vi "Harry_kane_home_use.vi"() -> ()   [LabVIEW 2013]
uses:
  <vilib>/vision/NI_Vision_Development_Module.lvlib
panel:
  out "appended array":cluster{"X":sgl, "Y":sgl}[](array[cluster])
  out "Pitch Image":T1(plugin-control)
  out "Player Position Pixels":dbl[][](array[numeric])
  out "Puck position pixels":dbl[][](array[numeric])
  out "Player Array From Reference":dbl[][](array[numeric])
  out "Puck Array From Reference":dbl[][](array[numeric])
  in  "Calibrate":bool
  out "Binary":T1(plugin-control)
  out "Histogram":T2(graph)
  out "Image in":T1(plugin-control)
  in  "Stop":bool
  in  "Capture image":bool
  out "Calibrated":T1(plugin-control)
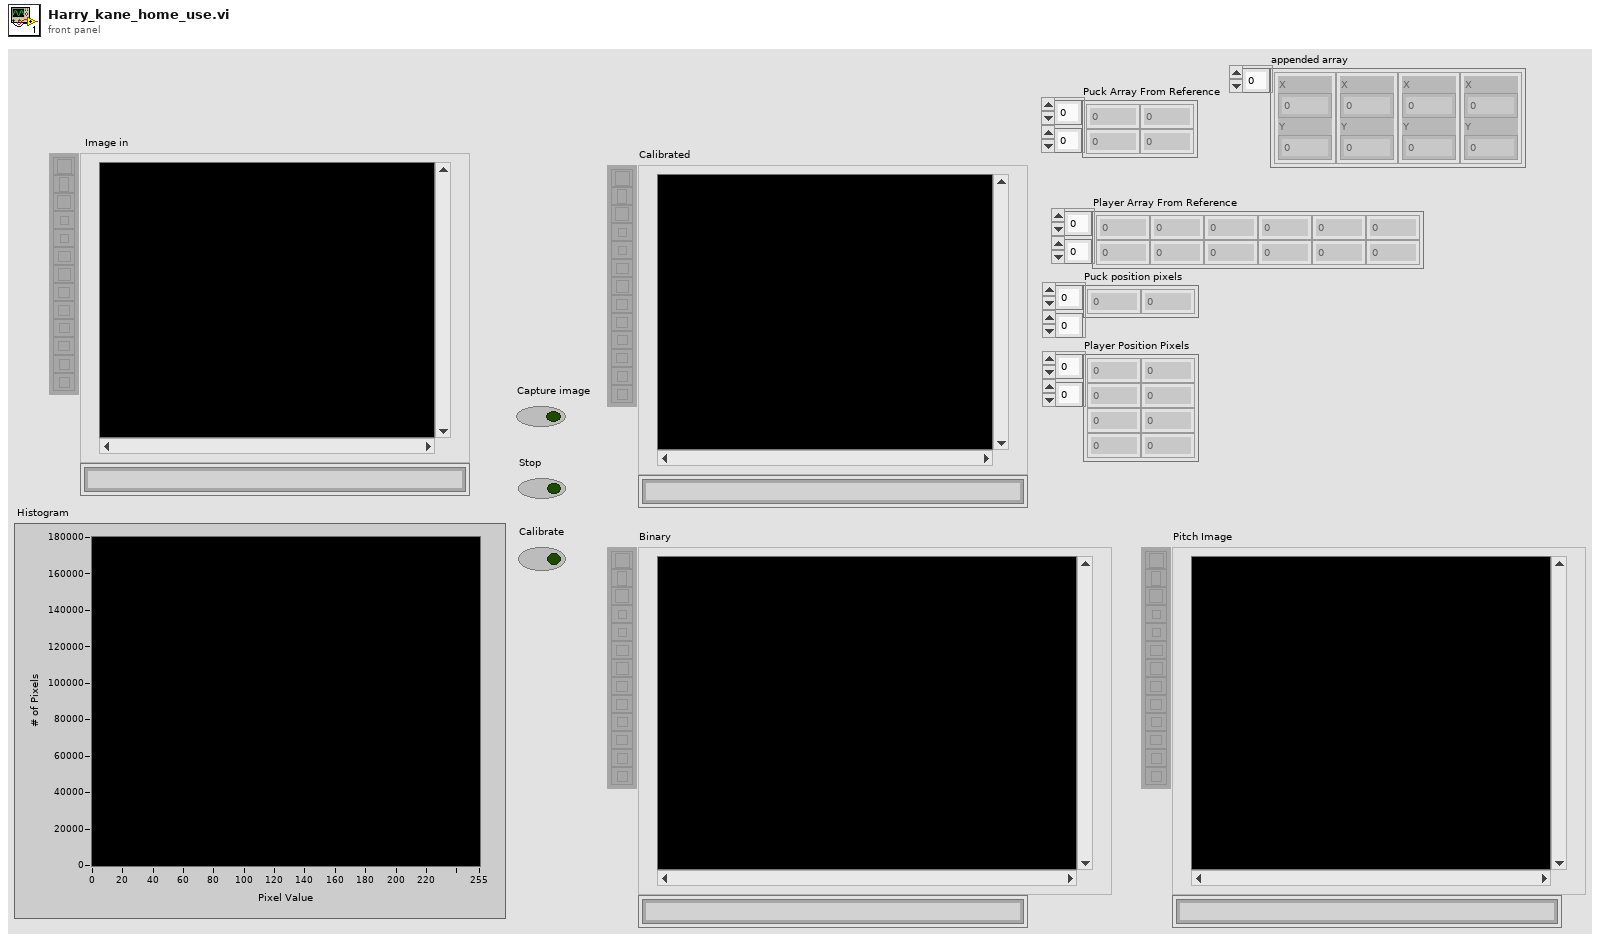
[diagram p1: front panel]
types:
  T1 = typedef "IMAQ Image.ctl" = refnum<image>
  T2 = cluster{"Starting Value":sgl, "Incremental Value":sgl, "Histogram":u32[]}
  T3 = typedef "Image Type" = u32
  T4 = cluster{"Point1 (Pixels)":cluster{"X":sgl, "Y":sgl}, "Point2 (Pixels)":cluster{"X":sgl, "Y":sgl}, "Point1 (Real-World)":cluster{"X":sgl, "Y":sgl}, "Point2 (Real-World)":cluster{"X":sgl, "Y":sgl}, "Angle (Pixel)":dbl, "Angle (Real-World)":dbl, "Score":dbl, "Straightness":dbl, "Average SNR (db)":dbl, "Calibration Valid":bool}
  T5 = cluster{"Start Point":cluster{"X":sgl, "Y":sgl}, "End Point":cluster{"X":sgl, "Y":sgl}, "Length":dbl, "Orientation":dbl, "Score":dbl}[]
  T6 = cluster{"Point1 (Pixels)":cluster{"X":sgl, "Y":sgl}, "Point2 (Pixels)":cluster{"X":sgl, "Y":sgl}}
  T7 = cluster{"Start Point":cluster{"X":sgl, "Y":sgl}, "End Point":cluster{"X":sgl, "Y":sgl}, "Length":dbl, "Orientation":dbl, "Score":dbl}
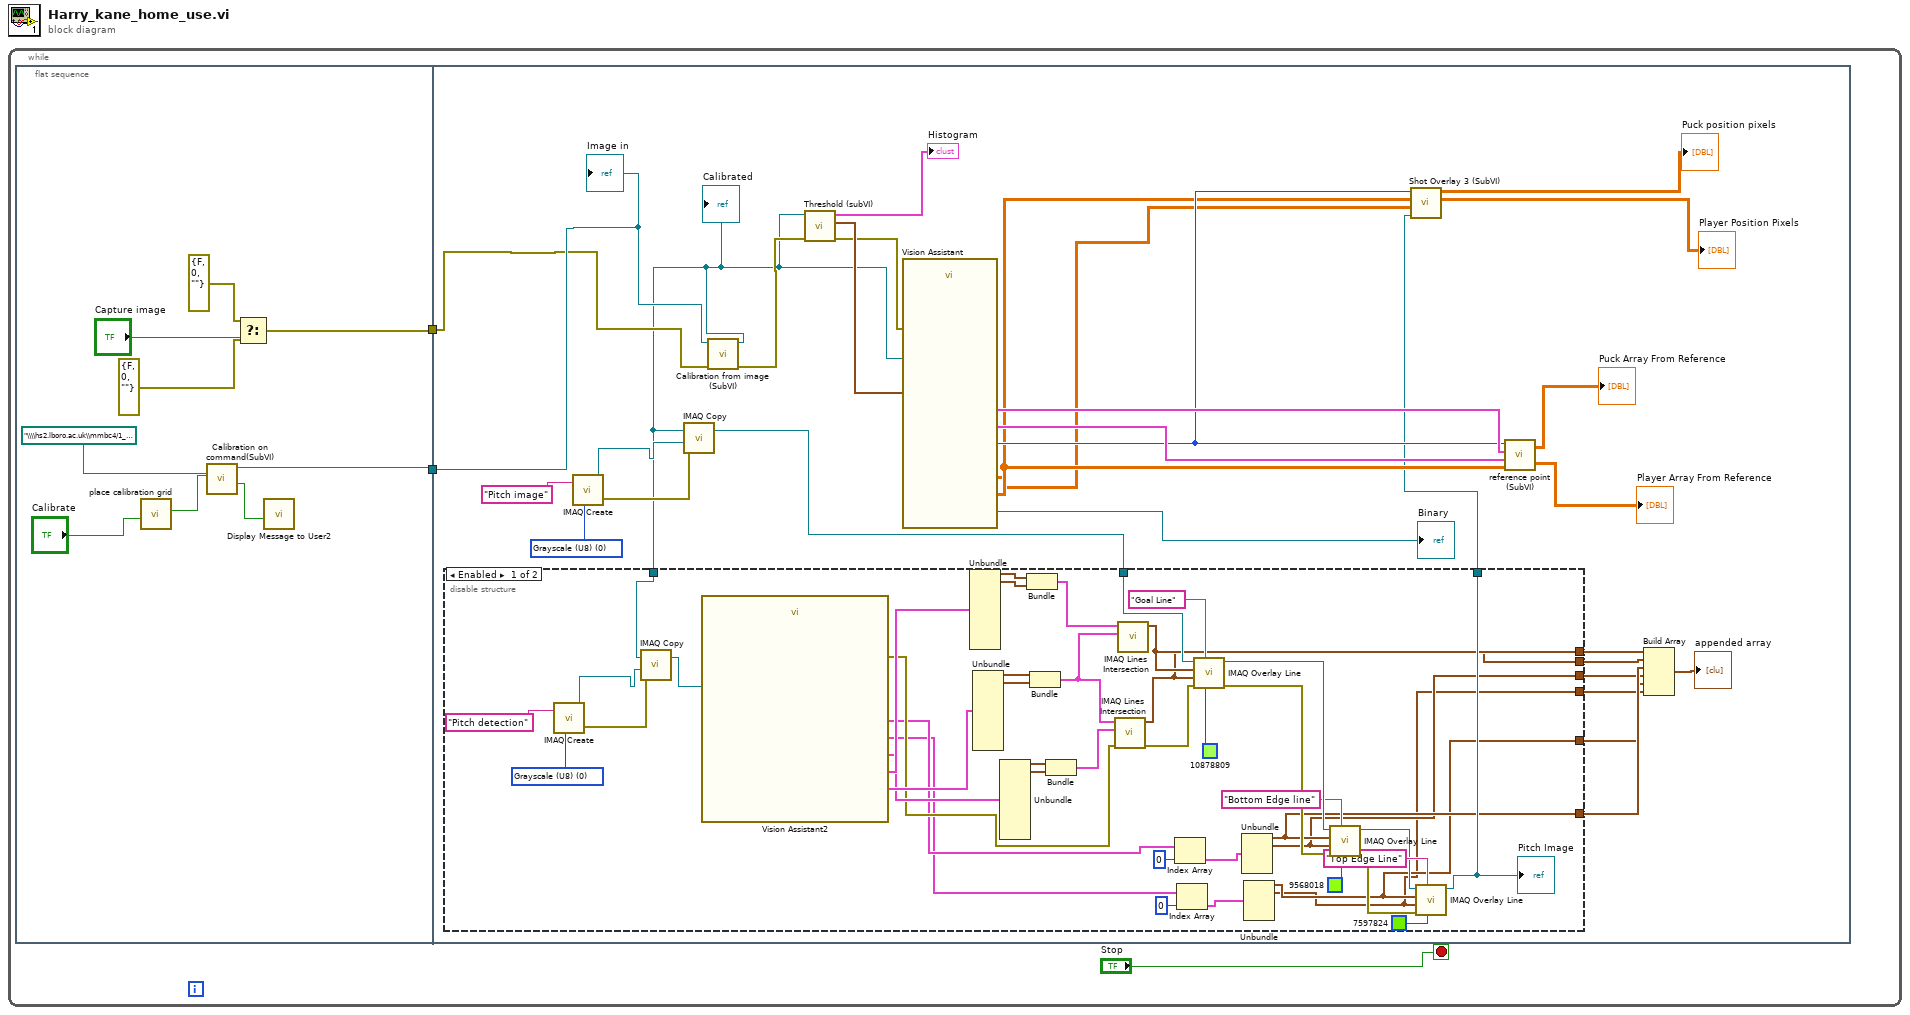
[diagram p0: block diagram]
diagram:
  n1 = while {
    stop <- "Stop" stop-if-true
    n2 = flat-sequence {
      tunnel: [w9] -> w2
      tunnel: [w7] -> w1
      tunnel: w2 -> [w37]
      tunnel: w1 -> [w38]
      frame #0 {
        n3 = call "place calibration grid"("Enable"="Calibrate") -> ("OK"=w5:bool)  [unwired: 9 in, 1 out]
        n4 = call "Calibration on command(SubVI).vi"("Calibrate"=w5, "File Path (Image Calibration 1)"=path "\\\\hs2.lboro.ac.uk\\mmbc4/1_Univesity Work/Mechatronics/Machine Vision/2.0_Harry_kane/Auto_calibration.png") -> ("Boolean"=w4:bool, "Refnum out"=w7:T1)  [unwired: 7 in, 1 out]
        n5 = Select(t=errorcluster {"status"=FALSE, "code"=0, "source"=""} ("error in"), s="Capture image", f=errorcluster {"status"=FALSE, "code"=0, "source"=""} ("error in")) -> (s? t:f=w9:errorcluster)
        n6 = call "Display Message to User2"("Enable"=w4) -> ()  [unwired: 9 in, 2 out]
      }
      frame #1 {
        w25 = T3 0 items=["Grayscale (U8)", "Grayscale (I16)", "Grayscale (SGL)", "Complex (CSG)", "RGB (U32)", "HSL (U32)", "RGB (U64)", "Grayscale (U16)"] ("Image Type")
        n7 = call "IMAQ Create"("Image Name"="Pitch image", "Image Type"=w25) -> ("New Image"=w27:T1, "error out"=w26:errorcluster)  [unwired: 3 in]
        n8 = call "Calibration from image (SubVI).vi"("error in (no error)"=w37, "Refnum in"=w38) -> ("error out"=w36:errorcluster, "Refnum out"=w23:T1)  [unwired: 8 in]
        "Calibrated" <- w23
        n9 = call "IMAQ Copy"("error in (no error)"=w26, "Image Dst"=w27, "Image Src"=w23) -> ("Image Dst Out"=w22:T1)  [unwired: 3 in, 1 out]
        n10 = disable-structure shown="Enabled" {
          disable-tunnel: w23 -> [w86 _]
          disable-tunnel: w22 -> [w64 _]
          disable-tunnel: [w49 _] -> w20
          disable-tunnel: [w48 _] -> w19
          disable-tunnel: [w47 _] -> w18
          disable-tunnel: [w46 _] -> w17
          disable-tunnel: [w45 _] -> w16
          disable-tunnel: [w44 _] -> w15
          disable-tunnel: [w43 _] -> w14
          frame Enabled {
            w83 = T3 0 items=["Grayscale (U8)", "Grayscale (I16)", "Grayscale (SGL)", "Complex (CSG)", "RGB (U32)", "HSL (U32)", "RGB (U64)", "Grayscale (U16)"] ("Image Type")
            n11 = call "IMAQ Create"("Image Name"="Pitch detection", "Image Type"=w83) -> ("New Image"=w85:T1, "error out"=w84:errorcluster)  [unwired: 3 in]
            n12 = call "IMAQ Copy"("error in (no error)"=w84, "Image Dst"=w85, "Image Src"=w86) -> ("Image Dst Out"=w69:T1)  [unwired: 3 in, 1 out]
            n13 = call "Vision Assistant2"("Image In"=w69) -> ("Straight Edge (Top goal edge)"=w73:T4, "Lines (Bottom Edge Detection)"=w63:T5, "Lines (Top Edge Detection)"=w56:T5, "Straight Edge (Bottom goal edge)"=w81:T4, "Straight Edge (Goal Line)"=w77:T4, "error out"=w68:errorcluster)  [unwired: 20 in, 1 out]
            n14 = Unbundle(w81) -> ("Point1 (Pixels)"=w80:cluster{"X":sgl, "Y":sgl}, "Point2 (Pixels)"=w79:cluster{"X":sgl, "Y":sgl})  [unwired: 8 out]
            n15 = Unbundle(w77) -> ("Point1 (Pixels)"=w76:cluster{"X":sgl, "Y":sgl}, "Point2 (Pixels)"=w75:cluster{"X":sgl, "Y":sgl})  [unwired: 8 out]
            n16 = Unbundle(w73) -> ("Point1 (Pixels)"=w72:cluster{"X":sgl, "Y":sgl}, "Point2 (Pixels)"=w71:cluster{"X":sgl, "Y":sgl})  [unwired: 8 out]
            n17 = Bundle("Point1 (Pixels)"=w80, "Point2 (Pixels)"=w79) -> (w78:T6)  [unwired: 1 in]
            n18 = Bundle("Point1 (Pixels)"=w76, "Point2 (Pixels)"=w75) -> (w74:T6)  [unwired: 1 in]
            n19 = Bundle("Point1 (Pixels)"=w72, "Point2 (Pixels)"=w71) -> (w70:T6)  [unwired: 1 in]
            n20 = call "IMAQ Lines Intersection"("error in (no error)"=w68, "Line 2"=w70, "Line 1"=w74) -> ("error out"=w67:errorcluster, "Intersection Point"=w47:cluster{"X":sgl, "Y":sgl})  [unwired: 6 in, 1 out]
            n21 = call "IMAQ Lines Intersection"("Line 2"=w74, "Line 1"=w78) -> ("Intersection Point"=w48:cluster{"X":sgl, "Y":sgl})  [unwired: 7 in, 2 out]
            n22 = Index Array(array=w63, index=0) -> (element=w61:T7)
            n23 = Index Array(array=w56, index=0) -> (element=w54:T7)
            n24 = call "IMAQ Overlay Line"("Color"=u32 10878809, "Group"="Goal Line", "error in (no error)"=w67, "End Point"=w47, "Start Point"=w48, "Image"=w64) -> ("error out"=w60:errorcluster, "Image Out"=w59:T1)  [unwired: 4 in]
            n25 = Unbundle(w61) -> ("Start Point"=w46:cluster{"X":sgl, "Y":sgl}, "End Point"=w45:cluster{"X":sgl, "Y":sgl})  [unwired: 3 out]
            n26 = Unbundle(w54) -> ("Start Point"=w44:cluster{"X":sgl, "Y":sgl}, "End Point"=w43:cluster{"X":sgl, "Y":sgl})  [unwired: 3 out]
            n27 = call "IMAQ Overlay Line"("Color"=u32 9568018, "Group"="Bottom Edge line", "error in (no error)"=w60, "End Point"=w45, "Start Point"=w46, "Image"=w59) -> ("error out"=w53:errorcluster, "Image Out"=w50:T1)  [unwired: 4 in]
            n28 = call "IMAQ Overlay Line"("Color"=u32 7597824, "Group"="Top Edge Line", "error in (no error)"=w53, "End Point"=w43, "Start Point"=w44, "Image"=w50) -> ("Image Out"=w49:T1)  [unwired: 4 in, 1 out]
            "Pitch Image" <- w49
          }
          frame Disabled {
          }
        }
        n29 = call "Threshold (subVI).vi"("error in (no error)"=w36, "Image  in"=w23) -> ("error out"=w35:errorcluster, "Cluster"=w42:cluster{sgl, "element":sgl}, "Histogram"=→"Histogram":T2)  [unwired: 7 in]
        n30 = call "Vision Assistant"("Image In"=w23, "Range (Threshold 1)"=w42, "error in"=w35) -> ("Image Out"=→"Binary":T1, "Particle Measurements (Real-World) (Particle Analysis 1)"=w31:dbl[][], "Particle Measurements (Pixels) (Particle Analysis 1)"=w30:dbl[][], "Straight Edge (Find Straight Edge 1)"=w40:T4, "Straight Edge (Find Straight Edge 2)"=w39:T4, "Nb Circles (Circle Detection 1)"=w32:i32)  [unwired: 17 in, 2 out]
        n31 = call "Shot Overlay 3 (SubVI).vi"("Image Out"=w20, "Particle Measurements (Pixels) (Particle Analysis 1)"=w30, "Particle Measurements (Real-World) (Particle Analysis 1)"=w31, "Nb Circles (Circle Detection 1)"=w32) -> ("Player Position Pixels"=→"Player Position Pixels":dbl[][], "Puck position pixels"=→"Puck position pixels":dbl[][])  [unwired: 4 in]
        n32 = call "reference point (SubVI).vi"("Nb Circles (Circle Detection 1)"=w32, "Straight Edge (Find Straight Edge 1)"=w40, "Straight Edge (Find Straight Edge 2)"=w39, "Particle Measurements (Real-World) (Particle Analysis 1)"=w31) -> ("Puck X, Y co-ordinates"=→"Puck Array From Reference":dbl[][], "Player X, Y co-ordinates"=→"Player Array From Reference":dbl[][])  [unwired: 1 in]
        n33 = Build Array(w19, w18, w17, w16, w15, w14) -> (→"appended array":cluster{"X":sgl, "Y":sgl}[])
        "Image in" <- w38
      }
    }
  }
